vi "3.register-while-loop.vi"() -> ()   [LabVIEW 2010]
panel:
  out "x+y =":i32
  out "Iteration-no":dbl
  in  "stop":bool
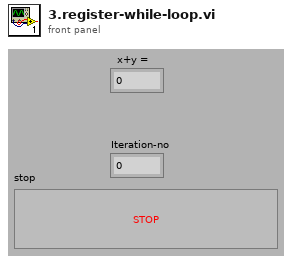
[diagram p1: front panel]
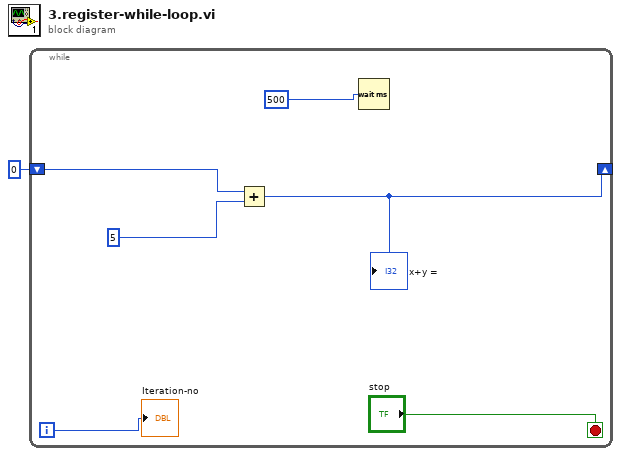
[diagram p0: block diagram]
diagram:
  n1 = while {
    shift-right: [w3] -> _
    shift-left: 0 -> [w4]
    i -> [w6]
    stop <- "stop" stop-if-true
    n2 = Add(x=w4, y=5) -> (x+y=w3:i32)
    "x+y =" <- w3
    n3 = Wait (ms)(milliseconds to wait=500) -> ()  [unwired: 1 out]
    "Iteration-no" <- w6
  }
